vi "eMICs response.vi"(8 "error in":errorcluster, 10 "eMIC response":T1[](array[typedef]), 11 "Module ID":i32=-1) -> (0 "error out":errorcluster)   [LabVIEW 2018, in "CE14  Module.lvlib"]
doc: "When complete Reading, report value to Caller\n_____\nCreated using DQMH Event Scripter 6.0.0.122."
uses:
  CE14  Module.lvlib
  Instrument Drivers/LVdriver_CE14(eMIC)/type defs/CE14.data.ctl
  eMICs response Argument--cluster.ctl
  Instrument Drivers/LVdriver_CE14(eMIC)/CE14_eMIC.lvlib
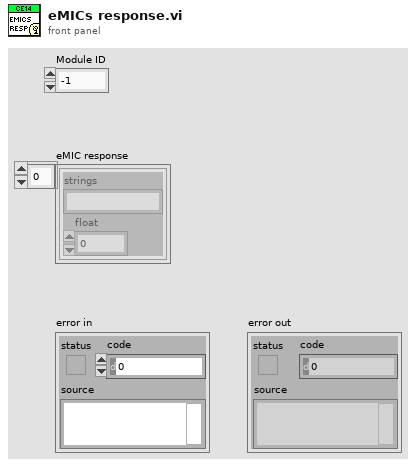
[diagram p1: front panel]
types:
  T1 = typedef "CE14_eMIC.lvlib/CE14.data.ctl" = cluster{"strings":string, "float":dbl}
  T2 = typedef "CE14  Module.lvlib/eMICs response Argument--cluster.ctl" = cluster{"Module ID":i32, "eMIC response":T1[]}
  T3 = typedef "CE14  Module.lvlib/Broadcast Events--cluster.ctl" = cluster{"Module Did Init":refnum<user-event>, "Status Updated":refnum<user-event>, "Error Reported":refnum<user-event>, "Module Did Stop":refnum<user-event>, "Update Module Execution Status":refnum<user-event>, "eMICs response":refnum<user-event>}
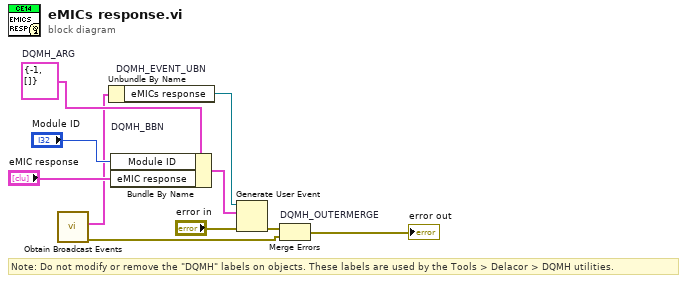
[diagram p0: block diagram]
diagram:
  w5 = T2 {"Module ID"=-1, "eMIC response"=[]}  # DQMH_ARG
  # "Note: Do not modify or remove the \"DQMH\" labels on objects. These labels are used by the Tools > Delacor > DQMH utilities."
  n1 = call "Obtain Broadcast Events.vi"() -> ("error out"=w2:errorcluster, "CE14  Module Broadcast Events"=w1:T3)  [unwired: 10 in]
  n2 = Unbundle By Name "DQMH_EVENT_UBN"(w1) -> ("eMICs response"=w7:refnum<user-event>)
  n3 = Bundle By Name "DQMH_BBN"(cluster=w5, "Module ID"="Module ID", "eMIC response"="eMIC response") -> (w8:T2)
  n4 = Generate User Event(user event=w7, event data cluster=w8, error in="error in") -> (error out=w6:errorcluster)  [unwired: 1 in, 1 out]
  n5 = Merge Errors "DQMH_OUTERMERGE"(w6, w2) -> (→"error out":errorcluster)
